vi "test add event.vi"() -> ()   [LabVIEW 2019, in "Logger.lvclass"]
uses:
  Logger_class/Logger.lvclass
  Logger_class/EventData.ctl
  TypeDef/AlarmType.ctl
panel:
  out "Set 2":set{string}(c389)
  out "Set":set{string}(c389)
  in  "new events 2":T1[](array[typedef])=[{"obj_tag"="AI0", "event_tag"="AI0.OUT_OF_RANGE_MIN", "Description"="Уровень  масла (НС очистки и охлаждения). Вне диапазона (низкий уровень)", "ALARM TYPE"=enum."Alarm", "Value DBL"=-0.000720119846917187, "Value INT"=1, "Value STR"="Alarm", "Time Stamp"=timestamp(3831935304.696055 s since 1904-01-01)}, {"obj_tag"="AI1", "event_tag"="AI1.OUT_OF_RANGE_MIN", "Description"="Уровень масла (НС подачи масла). Вне диапазона (низкий уровень)", "ALARM TYPE"=enum."Alarm", "Value DBL"=-0.0006009105573664057, "Value INT"=1, "Value STR"="Alarm", "Time Stamp"=timestamp(3831935304.696158 s since 1904-01-01)}, {"obj_tag"="AI2", "event_tag"="AI2.OUT_OF_RANGE_MIN", "Description"="Температура масла (НС очистки и охлаждения). Вне диапазона (низкий уровень)", "ALARM TYPE"=enum."Alarm", "Value DBL"=-0.00046664569044360226, "Value INT"=1, "Value STR"="Alarm", "Time Stamp"=timestamp(3831935304.696252 s since 1904-01-01)}, {"obj_tag"="AI3", "event_tag"="AI3.OUT_OF_RANGE_MIN", "Description"="Температура масла (НС подачи масла). Вне диапазона (низкий уровень)", "ALARM TYPE"=enum."Alarm", "Value DBL"=-0.0006016054301681914, "Value INT"=1, "Value STR"="Alarm", "Time Stamp"=timestamp(3831935304.696363 s since 1904-01-01)}, {"obj_tag"="AI4", "event_tag"="AI4.OUT_OF_RANGE_MIN", "Description"="Обратная связь от клапана регулировки низкого давления . Вне диапазона (низкий уровень)", "ALARM TYPE"=enum."Alarm", "Value DBL"=-0.00044842458141900095, "Value INT"=1, "Value STR"="Alarm", "Time Stamp"=timestamp(3831935304.696455 s since 1904-01-01)}, {"obj_tag"="AI5", "event_tag"="AI5.OUT_OF_RANGE_MIN", "Description"="Давление после насоса ВД. Вне диапазона (низкий уровень)", "ALARM TYPE"=enum."Alarm", "Value DBL"=-0.0004746753317086808, "Value INT"=1, "Value STR"="Alarm", "Time Stamp"=timestamp(3831935304.696545 s since 1904-01-01)}, {"obj_tag"="AI6", "event_tag"="AI6.OUT_OF_RANGE_MIN", "Description"="Давление в образце. Вне диапазона (низкий уровень)", "ALARM TYPE"=enum."Alarm", "Value DBL"=-0.0004625536617219757, "Value INT"=1, "Value STR"="Alarm", "Time Stamp"=timestamp(3831935304.696636 s since 1904-01-01)}, {"obj_tag"="AI7", "event_tag"="AI7.OUT_OF_RANGE_MIN", "Description"="Давление в камере. Вне диапазона (низкий уровень)", "ALARM TYPE"=enum."Alarm", "Value DBL"=-0.0004948266429604644, "Value INT"=1, "Value STR"="Alarm", "Time Stamp"=timestamp(3831935304.696729 s since 1904-01-01)}, {"obj_tag"="AI8", "event_tag"="AI8.OUT_OF_RANGE_MIN", "Description"="Давление  в  линии подачи воздуха в  БПВ. Вне диапазона (низкий уровень)", "ALARM TYPE"=enum."Alarm", "Value DBL"=-0.0005392985022747455, "Value INT"=1, "Value STR"="Alarm", "Time Stamp"=timestamp(3831935304.696866 s since 1904-01-01)}, {"obj_tag"="AI9", "event_tag"="AI9.OUT_OF_RANGE_MIN", "Description"="Давление  в  линии подачи воздуха после БПВ. Вне диапазона (низкий уровень)", "ALARM TYPE"=enum."Alarm", "Value DBL"=-0.00044981432702257226, "Value INT"=1, "Value STR"="Alarm", "Time Stamp"=timestamp(3831935304.69696 s since 1904-01-01)}, {"obj_tag"="DI0", "event_tag"="DI0.DI", "Description"="Автомат QF1", "ALARM TYPE"=enum."Normal", "Value DBL"=1.0, "Value INT"=1, "Value STR"="True", "Time Stamp"=timestamp(3831935304.697038 s since 1904-01-01)}, {"obj_tag"="DI1", "event_tag"="DI1.DI", "Description"="Автомат QF2", "ALARM TYPE"=enum."Normal", "Value DBL"=1.0, "Value INT"=1, "Value STR"="True", "Time Stamp"=timestamp(3831935304.697049 s since 1904-01-01)}, {"obj_tag"="DI2", "event_tag"="DI2.DI", "Description"="Автомат QF3", "ALARM TYPE"=enum."Normal", "Value DBL"=1.0, "Value INT"=1, "Value STR"="True", "Time Stamp"=timestamp(3831935304.697056 s since 1904-01-01)}, {"obj_tag"="DI3", "event_tag"="DI3.DI", "Description"="Автомат QF4", "ALARM TYPE"=enum."Normal", "Value DBL"=1.0, "Value INT"=1, "Value STR"="True", "Time Stamp"=timestamp(3831935304.697061 s since 1904-01-01)}, {"obj_tag"="DI4", "event_tag"="DI4.DI", "Description"="Автомат QF5", "ALARM TYPE"=enum."Normal", "Value DBL"=1.0, "Value INT"=1, "Value STR"="True", "Time Stamp"=timestamp(3831935304.697067 s since 1904-01-01)}, {"obj_tag"="DI5", "event_tag"="DI5.DI", "Description"="Автомат QF6", "ALARM TYPE"=enum."Normal", "Value DBL"=1.0, "Value INT"=1, "Value STR"="True", "Time Stamp"=timestamp(3831935304.697073 s since 1904-01-01)}, {"obj_tag"="DI6", "event_tag"="DI6.DI", "Description"="Автомат QF7", "ALARM TYPE"=enum."Normal", "Value DBL"=1.0, "Value INT"=1, "Value STR"="True", "Time Stamp"=timestamp(3831935304.697079 s since 1904-01-01)}, {"obj_tag"="DI7", "event_tag"="DI7.DI", "Description"="Автомат QF8", "ALARM TYPE"=enum."Normal", "Value DBL"=1.0, "Value INT"=1, "Value STR"="True", "Time Stamp"=timestamp(3831935304.697137 s since 1904-01-01)}, {"obj_tag"="DI8", "event_tag"="DI8.DI", "Description"="Автомат QF9", "ALARM TYPE"=enum."Normal", "Value DBL"=1.0, "Value INT"=1, "Value STR"="True", "Time Stamp"=timestamp(3831935304.697145 s since 1904-01-01)}, {"obj_tag"="DI10", "event_tag"="DI10.DI", "Description"="Состояние БП [G1]", "ALARM TYPE"=enum."Normal", "Value DBL"=1.0, "Value INT"=1, "Value STR"="True", "Time Stamp"=timestamp(3831935304.697152 s since 1904-01-01)}, {"obj_tag"="DI11", "event_tag"="DI11.DI", "Description"="Состояние БП [G2]", "ALARM TYPE"=enum."Normal", "Value DBL"=1.0, "Value INT"=1, "Value STR"="True", "Time Stamp"=timestamp(3831935304.697158 s since 1904-01-01)}, {"obj_tag"="DI15", "event_tag"="DI15.DI", "Description"="Кнопка аварийной остановки [SB4]", "ALARM TYPE"=enum."Normal", "Value DBL"=1.0, "Value INT"=1, "Value STR"="True", "Time Stamp"=timestamp(3831935304.697164 s since 1904-01-01)}, {"obj_tag"="STAND", "event_tag"="DO5", "Description"="Клапан KP6 Y29.1 33.7", "ALARM TYPE"=enum."Normal", "Value DBL"=1.0, "Value INT"=1, "Value STR"="True", "Time Stamp"=timestamp(3831935304.697175 s since 1904-01-01)}, {"obj_tag"="STAND", "event_tag"="DO6", "Description"="Клапан KP7 Y29.2 33.8 ", "ALARM TYPE"=enum."Normal", "Value DBL"=1.0, "Value INT"=1, "Value STR"="True", "Time Stamp"=timestamp(3831935304.697185 s since 1904-01-01)}, {"obj_tag"="STAND", "event_tag"="DO7", "Description"="Клапан KP8 Y29.3 33.9 ", "ALARM TYPE"=enum."Normal", "Value DBL"=1.0, "Value INT"=1, "Value STR"="True", "Time Stamp"=timestamp(3831935304.697191 s since 1904-01-01)}, {"obj_tag"="STAND", "event_tag"="DO8", "Description"="Клапан KP9 Y29.4  33.12 ", "ALARM TYPE"=enum."Normal", "Value DBL"=1.0, "Value INT"=1, "Value STR"="True", "Time Stamp"=timestamp(3831935304.697197 s since 1904-01-01)}, {"obj_tag"="STAND", "event_tag"="DO9", "Description"="Клапан KP10 Y29.5 33.1 ", "ALARM TYPE"=enum."Normal", "Value DBL"=1.0, "Value INT"=1, "Value STR"="True", "Time Stamp"=timestamp(3831935304.697212 s since 1904-01-01)}, {"obj_tag"="STAND", "event_tag"="DO10", "Description"="Клапан KP11 Y29.6 33.2 ", "ALARM TYPE"=enum."Normal", "Value DBL"=1.0, "Value INT"=1, "Value STR"="True", "Time Stamp"=timestamp(3831935304.697243 s since 1904-01-01)}, {"obj_tag"="STAND", "event_tag"="DO11", "Description"="Клапан KP12 Y29.7  33.13 ", "ALARM TYPE"=enum."Normal", "Value DBL"=1.0, "Value INT"=1, "Value STR"="True", "Time Stamp"=timestamp(3831935304.697255 s since 1904-01-01)}, {"obj_tag"="STAND", "event_tag"="DO12", "Description"="Клапан KP13 Y29.8  33.11 ", "ALARM TYPE"=enum."Normal", "Value DBL"=1.0, "Value INT"=1, "Value STR"="True", "Time Stamp"=timestamp(3831935304.697262 s since 1904-01-01)}, {"obj_tag"="STAND", "event_tag"="DO13", "Description"="Клапан KP14 Y29.9 33.10 ", "ALARM TYPE"=enum."Normal", "Value DBL"=1.0, "Value INT"=1, "Value STR"="True", "Time Stamp"=timestamp(3831935304.697268 s since 1904-01-01)}, {"obj_tag"="STAND", "event_tag"="DO14", "Description"="Клапан KP15 Y29.10  33.6 ", "ALARM TYPE"=enum."Normal", "Value DBL"=1.0, "Value INT"=1, "Value STR"="True", "Time Stamp"=timestamp(3831935304.697274 s since 1904-01-01)}, {"obj_tag"="STAND", "event_tag"="DO15", "Description"="Клапан KP16 Y29.11  33.5 ", "ALARM TYPE"=enum."Normal", "Value DBL"=1.0, "Value INT"=1, "Value STR"="True", "Time Stamp"=timestamp(3831935304.697279 s since 1904-01-01)}, {"obj_tag"="STAND", "event_tag"="DO16", "Description"="Клапан KP17 Y29.12  33.4 ", "ALARM TYPE"=enum."Normal", "Value DBL"=1.0, "Value INT"=1, "Value STR"="True", "Time Stamp"=timestamp(3831935304.697374 s since 1904-01-01)}, {"obj_tag"="STAND", "event_tag"="DO17", "Description"="Клапан KP18 Y29.13 33.3 ", "ALARM TYPE"=enum."Normal", "Value DBL"=1.0, "Value INT"=1, "Value STR"="True", "Time Stamp"=timestamp(3831935304.697383 s since 1904-01-01)}, {"obj_tag"="STAND", "event_tag"="DO19", "Description"="Драйверы KP20", "ALARM TYPE"=enum."Normal", "Value DBL"=1.0, "Value INT"=1, "Value STR"="True", "Time Stamp"=timestamp(3831935304.69739 s since 1904-01-01)}, {"obj_tag"="STAND", "event_tag"="DO24", "Description"="Сигнал остановки шагового драйвера 1", "ALARM TYPE"=enum."Normal", "Value DBL"=1.0, "Value INT"=1, "Value STR"="True", "Time Stamp"=timestamp(3831935304.697397 s since 1904-01-01)}, {"obj_tag"="STAND", "event_tag"="DO25", "Description"="Сигнал остановки шагового драйвера 2", "ALARM TYPE"=enum."Normal", "Value DBL"=1.0, "Value INT"=1, "Value STR"="True", "Time Stamp"=timestamp(3831935304.697403 s since 1904-01-01)}, {"obj_tag"="NV1", "event_tag"="NV1.OL", "Description"="Игольчатый клапан плавного спуска (образец). Состояние разомкнутой нагрузки", "ALARM TYPE"=enum."Normal", "Value DBL"=0.0, "Value INT"=0, "Value STR"="Normal", "Time Stamp"=timestamp(3831935304.707156 s since 1904-01-01)}, {"obj_tag"="NV1", "event_tag"="NV1.TF", "Description"="Игольчатый клапан плавного спуска (образец). Предупреждения о перегреве и отключения при перегреве", "ALARM TYPE"=enum."Normal", "Value DBL"=0.0, "Value INT"=0, "Value STR"="Normal", "Time Stamp"=timestamp(3831935304.707491 s since 1904-01-01)}, {"obj_tag"="NV1", "event_tag"="NV1.STL", "Description"="Игольчатый клапан плавного спуска (образец). Состояние остановки двигателя", "ALARM TYPE"=enum."Normal", "Value DBL"=0.0, "Value INT"=0, "Value STR"="Normal", "Time Stamp"=timestamp(3831935304.707583 s since 1904-01-01)}, {"obj_tag"="NV1", "event_tag"="NV1.OCP", "Description"="Игольчатый клапан плавного спуска (образец). Перегрузка по току", "ALARM TYPE"=enum."Normal", "Value DBL"=0.0, "Value INT"=0, "Value STR"="Normal", "Time Stamp"=timestamp(3831935304.707645 s since 1904-01-01)}, {"obj_tag"="NV1", "event_tag"="NV1.CPUV", "Description"="Игольчатый клапан плавного спуска (образец). charge pump undervoltage", "ALARM TYPE"=enum."Normal", "Value DBL"=0.0, "Value INT"=0, "Value STR"="Normal", "Time Stamp"=timestamp(3831935304.707712 s since 1904-01-01)}, {"obj_tag"="NV1", "event_tag"="NV1.UVLO", "Description"="Игольчатый клапан плавного спуска (образец). Пониженное напряжение питания", "ALARM TYPE"=enum."Normal", "Value DBL"=0.0, "Value INT"=0, "Value STR"="Normal", "Time Stamp"=timestamp(3831935304.707769 s since 1904-01-01)}, {"obj_tag"="NV1", "event_tag"="NV1.SPI_ERROR", "Description"="Игольчатый клапан плавного спуска (образец). Ошибки протокола SPI", "ALARM TYPE"=enum."Normal", "Value DBL"=0.0, "Value INT"=0, "Value STR"="Normal", "Time Stamp"=timestamp(3831935304.707827 s since 1904-01-01)}, {"obj_tag"="NV1", "event_tag"="NV1.Fault", "Description"="Игольчатый клапан плавного спуска (образец). Общая неисправность", "ALARM TYPE"=enum."Normal", "Value DBL"=0.0, "Value INT"=0, "Value STR"="Normal", "Time Stamp"=timestamp(3831935304.707885 s since 1904-01-01)}, {"obj_tag"="NV1", "event_tag"="NV1.INIT_ERROR", "Description"="Игольчатый клапан плавного спуска (образец). Ошибка инициализации", "ALARM TYPE"=enum."Normal", "Value DBL"=0.0, "Value INT"=0, "Value STR"="Normal", "Time Stamp"=timestamp(3831935304.707946 s since 1904-01-01)}, {"obj_tag"="NV1", "event_tag"="NV1.MB_ERROR", "Description"="Игольчатый клапан плавного спуска (образец). Ошибка подключения (модбас)", "ALARM TYPE"=enum."Normal", "Value DBL"=0.0, "Value INT"=0, "Value STR"="Normal", "Time Stamp"=timestamp(3831935304.707986 s since 1904-01-01)}, {"obj_tag"="NV1", "event_tag"="NV1.ST", "Description"="Игольчатый клапан плавного спуска (образец). Состояние", "ALARM TYPE"=enum."Normal", "Value DBL"=0.0, "Value INT"=0, "Value STR"="IDLE", "Time Stamp"=timestamp(3831935304.708018 s since 1904-01-01)}, {"obj_tag"="M22", "event_tag"="M22.UNPLANNED_TURN_OFF", "Description"="Двигатель охлаждения. Выключение без команды", "ALARM TYPE"=enum."Normal", "Value DBL"=0.0, "Value INT"=0, "Value STR"="Normal", "Time Stamp"=timestamp(3831935304.70986 s since 1904-01-01)}, {"obj_tag"="M12", "event_tag"="M12.UNPLANNED_TURN_OFF", "Description"="Двигатель перекачки. Выключение без команды", "ALARM TYPE"=enum."Normal", "Value DBL"=0.0, "Value INT"=0, "Value STR"="Normal", "Time Stamp"=timestamp(3831935304.71006 s since 1904-01-01)}, {"obj_tag"="M21", "event_tag"="M21.UNPLANNED_TURN_OFF", "Description"="Двигатель подачи масла. Выключение без команды", "ALARM TYPE"=enum."Normal", "Value DBL"=0.0, "Value INT"=0, "Value STR"="Normal", "Time Stamp"=timestamp(3831935304.71022 s since 1904-01-01)}, {"obj_tag"="M22", "event_tag"="M22.AUTOMAT_ERROR", "Description"="Двигатель охлаждения. Выключен автомат", "ALARM TYPE"=enum."Normal", "Value DBL"=0.0, "Value INT"=0, "Value STR"="Normal", "Time Stamp"=timestamp(3831935304.710246 s since 1904-01-01)}, {"obj_tag"="M22", "event_tag"="M22.UNPLANNED_TURN_ON", "Description"="Двигатель охлаждения. Включение без команды", "ALARM TYPE"=enum."Normal", "Value DBL"=0.0, "Value INT"=0, "Value STR"="Normal", "Time Stamp"=timestamp(3831935304.710273 s since 1904-01-01)}, {"obj_tag"="M22", "event_tag"="M22.ON_EEROR", "Description"="Двигатель охлаждения. Ошибка включения", "ALARM TYPE"=enum."Normal", "Value DBL"=0.0, "Value INT"=0, "Value STR"="Normal", "Time Stamp"=timestamp(3831935304.710294 s since 1904-01-01)}, {"obj_tag"="M22", "event_tag"="M22.OFF_ERROR", "Description"="Двигатель охлаждения. Ошибка выключения", "ALARM TYPE"=enum."Normal", "Value DBL"=0.0, "Value INT"=0, "Value STR"="Normal", "Time Stamp"=timestamp(3831935304.710315 s since 1904-01-01)}, {"obj_tag"="M22", "event_tag"="M22.ST", "Description"="Двигатель охлаждения. Состояние", "ALARM TYPE"=enum."Normal", "Value DBL"=1.0, "Value INT"=1, "Value STR"="Off", "Time Stamp"=timestamp(3831935304.710339 s since 1904-01-01)}, {"obj_tag"="M12", "event_tag"="M12.AUTOMAT_ERROR", "Description"="Двигатель перекачки. Выключен автомат", "ALARM TYPE"=enum."Normal", "Value DBL"=0.0, "Value INT"=0, "Value STR"="Normal", "Time Stamp"=timestamp(3831935304.710367 s since 1904-01-01)}, {"obj_tag"="M12", "event_tag"="M12.UNPLANNED_TURN_ON", "Description"="Двигатель перекачки. Включение без команды", "ALARM TYPE"=enum."Normal", "Value DBL"=0.0, "Value INT"=0, "Value STR"="Normal", "Time Stamp"=timestamp(3831935304.710392 s since 1904-01-01)}, {"obj_tag"="M12", "event_tag"="M12.ON_EEROR", "Description"="Двигатель перекачки. Ошибка включения", "ALARM TYPE"=enum."Normal", "Value DBL"=0.0, "Value INT"=0, "Value STR"="Normal", "Time Stamp"=timestamp(3831935304.710413 s since 1904-01-01)}, {"obj_tag"="M12", "event_tag"="M12.OFF_ERROR", "Description"="Двигатель перекачки. Ошибка выключения", "ALARM TYPE"=enum."Normal", "Value DBL"=0.0, "Value INT"=0, "Value STR"="Normal", "Time Stamp"=timestamp(3831935304.710432 s since 1904-01-01)}, {"obj_tag"="M12", "event_tag"="M12.ST", "Description"="Двигатель перекачки. Состояние", "ALARM TYPE"=enum."Normal", "Value DBL"=1.0, "Value INT"=1, "Value STR"="Off", "Time Stamp"=timestamp(3831935304.710451 s since 1904-01-01)}, {"obj_tag"="M21", "event_tag"="M21.AUTOMAT_ERROR", "Description"="Двигатель подачи масла. Выключен автомат", "ALARM TYPE"=enum."Normal", "Value DBL"=0.0, "Value INT"=0, "Value STR"="Normal", "Time Stamp"=timestamp(3831935304.710473 s since 1904-01-01)}, {"obj_tag"="M21", "event_tag"="M21.UNPLANNED_TURN_ON", "Description"="Двигатель подачи масла. Включение без команды", "ALARM TYPE"=enum."Normal", "Value DBL"=0.0, "Value INT"=0, "Value STR"="Normal", "Time Stamp"=timestamp(3831935304.710492 s since 1904-01-01)}, {"obj_tag"="M21", "event_tag"="M21.ON_EEROR", "Description"="Двигатель подачи масла. Ошибка включения", "ALARM TYPE"=enum."Normal", "Value DBL"=0.0, "Value INT"=0, "Value STR"="Normal", "Time Stamp"=timestamp(3831935304.710516 s since 1904-01-01)}, {"obj_tag"="M21", "event_tag"="M21.OFF_ERROR", "Description"="Двигатель подачи масла. Ошибка выключения", "ALARM TYPE"=enum."Normal", "Value DBL"=0.0, "Value INT"=0, "Value STR"="Normal", "Time Stamp"=timestamp(3831935304.710727 s since 1904-01-01)}, {"obj_tag"="M21", "event_tag"="M21.ST", "Description"="Двигатель подачи масла. Состояние", "ALARM TYPE"=enum."Normal", "Value DBL"=1.0, "Value INT"=1, "Value STR"="Off", "Time Stamp"=timestamp(3831935304.71075 s since 1904-01-01)}, {"obj_tag"="VALVE_44_1", "event_tag"="VALVE_44_1.LIMITS_ERROR", "Description"="Клапан 44.1. Ошибочное состояние концевиков", "ALARM TYPE"=enum."Normal", "Value DBL"=0.0, "Value INT"=0, "Value STR"="Normal", "Time Stamp"=timestamp(3831935304.711082 s since 1904-01-01)}, {"obj_tag"="VALVE_44_1", "event_tag"="VALVE_44_1.UNPLANNED_CLOSE", "Description"="Клапан 44.1. Закрытие без команды", "ALARM TYPE"=enum."Normal", "Value DBL"=0.0, "Value INT"=0, "Value STR"="Normal", "Time Stamp"=timestamp(3831935304.711128 s since 1904-01-01)}, {"obj_tag"="VALVE_44_1", "event_tag"="VALVE_44_1.UNPLANNED_OPEN", "Description"="Клапан 44.1. Открытие без команды", "ALARM TYPE"=enum."Normal", "Value DBL"=0.0, "Value INT"=0, "Value STR"="Normal", "Time Stamp"=timestamp(3831935304.711153 s since 1904-01-01)}, {"obj_tag"="VALVE_44_1", "event_tag"="VALVE_44_1.OPEN_ERROR", "Description"="Клапан 44.1. Ошибка открытия", "ALARM TYPE"=enum."Normal", "Value DBL"=0.0, "Value INT"=0, "Value STR"="Normal", "Time Stamp"=timestamp(3831935304.71118 s since 1904-01-01)}, {"obj_tag"="VALVE_44_1", "event_tag"="VALVE_44_1.CLOSE_ERROR", "Description"="Клапан 44.1.Ошибка закрытия", "ALARM TYPE"=enum."Normal", "Value DBL"=0.0, "Value INT"=0, "Value STR"="Normal", "Time Stamp"=timestamp(3831935304.711201 s since 1904-01-01)}, {"obj_tag"="VALVE_44_1", "event_tag"="VALVE_44_1.ST", "Description"="Клапан 44.1. Состояние", "ALARM TYPE"=enum."Normal", "Value DBL"=0.0, "Value INT"=0, "Value STR"="Unknown", "Time Stamp"=timestamp(3831935304.711225 s since 1904-01-01)}, {"obj_tag"="VALVE_44_2", "event_tag"="VALVE_44_2.LIMITS_ERROR", "Description"="Клапан 44.2. Ошибочное состояние концевиков", "ALARM TYPE"=enum."Normal", "Value DBL"=0.0, "Value INT"=0, "Value STR"="Normal", "Time Stamp"=timestamp(3831935304.711441 s since 1904-01-01)}, {"obj_tag"="VALVE_44_2", "event_tag"="VALVE_44_2.UNPLANNED_CLOSE", "Description"="Клапан 44.2. Закрытие без команды", "ALARM TYPE"=enum."Normal", "Value DBL"=0.0, "Value INT"=0, "Value STR"="Normal", "Time Stamp"=timestamp(3831935304.711487 s since 1904-01-01)}, {"obj_tag"="VALVE_44_2", "event_tag"="VALVE_44_2.UNPLANNED_OPEN", "Description"="Клапан 44.2. Открытие без команды", "ALARM TYPE"=enum."Normal", "Value DBL"=0.0, "Value INT"=0, "Value STR"="Normal", "Time Stamp"=timestamp(3831935304.711512 s since 1904-01-01)}, {"obj_tag"="VALVE_44_2", "event_tag"="VALVE_44_2.OPEN_ERROR", "Description"="Клапан 44.2. Ошибка открытия", "ALARM TYPE"=enum."Normal", "Value DBL"=0.0, "Value INT"=0, "Value STR"="Normal", "Time Stamp"=timestamp(3831935304.711537 s since 1904-01-01)}, {"obj_tag"="VALVE_44_2", "event_tag"="VALVE_44_2.CLOSE_ERROR", "Description"="Клапан 44.2.Ошибка закрытия", "ALARM TYPE"=enum."Normal", "Value DBL"=0.0, "Value INT"=0, "Value STR"="Normal", "Time Stamp"=timestamp(3831935304.711557 s since 1904-01-01)}, {"obj_tag"="STAND", "event_tag"="ERROR_QF1", "Description"="Ошибка автомат QF1", "ALARM TYPE"=enum."Normal", "Value DBL"=0.0, "Value INT"=0, "Value STR"="Normal", "Time Stamp"=timestamp(3831935304.711661 s since 1904-01-01)}, {"obj_tag"="STAND", "event_tag"="ERROR_QF2", "Description"="Ошибка автомат QF2", "ALARM TYPE"=enum."Normal", "Value DBL"=0.0, "Value INT"=0, "Value STR"="Normal", "Time Stamp"=timestamp(3831935304.711695 s since 1904-01-01)}, {"obj_tag"="STAND", "event_tag"="ERROR_QF3", "Description"="Ошибка автомат QF3", "ALARM TYPE"=enum."Normal", "Value DBL"=0.0, "Value INT"=0, "Value STR"="Normal", "Time Stamp"=timestamp(3831935304.711716 s since 1904-01-01)}, {"obj_tag"="STAND", "event_tag"="ERROR_QF4", "Description"="Ошибка автомат QF4", "ALARM TYPE"=enum."Normal", "Value DBL"=0.0, "Value INT"=0, "Value STR"="Normal", "Time Stamp"=timestamp(3831935304.711732 s since 1904-01-01)}, {"obj_tag"="STAND", "event_tag"="ERROR_QF5", "Description"="Ошибка автомат QF5", "ALARM TYPE"=enum."Normal", "Value DBL"=0.0, "Value INT"=0, "Value STR"="Normal", "Time Stamp"=timestamp(3831935304.711748 s since 1904-01-01)}, {"obj_tag"="STAND", "event_tag"="ERROR_QF6", "Description"="Ошибка автомат QF6", "ALARM TYPE"=enum."Normal", "Value DBL"=0.0, "Value INT"=0, "Value STR"="Normal", "Time Stamp"=timestamp(3831935304.711763 s since 1904-01-01)}, {"obj_tag"="STAND", "event_tag"="ERROR_QF7", "Description"="Ошибка автомат QF7", "ALARM TYPE"=enum."Normal", "Value DBL"=0.0, "Value INT"=0, "Value STR"="Normal", "Time Stamp"=timestamp(3831935304.711784 s since 1904-01-01)}, {"obj_tag"="STAND", "event_tag"="ERROR_QF8", "Description"="Ошибка автомат QF8", "ALARM TYPE"=enum."Normal", "Value DBL"=0.0, "Value INT"=0, "Value STR"="Normal", "Time Stamp"=timestamp(3831935304.711801 s since 1904-01-01)}, {"obj_tag"="STAND", "event_tag"="ERROR_QF9", "Description"="Ошибка автомат QF9", "ALARM TYPE"=enum."Normal", "Value DBL"=0.0, "Value INT"=0, "Value STR"="Normal", "Time Stamp"=timestamp(3831935304.711817 s since 1904-01-01)}, {"obj_tag"="STAND", "event_tag"="ERROR_QF9_FCR", "Description"="Ошибка реле контроля фаз", "ALARM TYPE"=enum."Normal", "Value DBL"=0.0, "Value INT"=0, "Value STR"="Normal", "Time Stamp"=timestamp(3831935304.711834 s since 1904-01-01)}, {"obj_tag"="STAND", "event_tag"="ERROR_G1", "Description"="Ошибка БП G1", "ALARM TYPE"=enum."Normal", "Value DBL"=0.0, "Value INT"=0, "Value STR"="Normal", "Time Stamp"=timestamp(3831935304.711856 s since 1904-01-01)}, {"obj_tag"="STAND", "event_tag"="ERROR_G2", "Description"="Ошибка БП G2", "ALARM TYPE"=enum."Normal", "Value DBL"=0.0, "Value INT"=0, "Value STR"="Normal", "Time Stamp"=timestamp(3831935304.711872 s since 1904-01-01)}, {"obj_tag"="STAND", "event_tag"="ERROR_MOD_1_NI_9425", "Description"="ERROR_MOD_1_NI_9425", "ALARM TYPE"=enum."Normal", "Value DBL"=0.0, "Value INT"=0, "Value STR"="Normal", "Time Stamp"=timestamp(3831935304.712015 s since 1904-01-01)}, {"obj_tag"="STAND", "event_tag"="ERROR_MOD_2_NI_9477", "Description"="ERROR_MOD_2_NI_9477", "ALARM TYPE"=enum."Normal", "Value DBL"=0.0, "Value INT"=0, "Value STR"="Normal", "Time Stamp"=timestamp(3831935304.712038 s since 1904-01-01)}, {"obj_tag"="STAND", "event_tag"="ERROR_MOD_3_NI_9203", "Description"="ERROR_MOD_3_NI_9203", "ALARM TYPE"=enum."Normal", "Value DBL"=0.0, "Value INT"=0, "Value STR"="Normal", "Time Stamp"=timestamp(3831935304.712056 s since 1904-01-01)}, {"obj_tag"="STAND", "event_tag"="ERROR_MOD_4_NI_9203", "Description"="ERROR_MOD_4_NI_9203", "ALARM TYPE"=enum."Normal", "Value DBL"=0.0, "Value INT"=0, "Value STR"="Normal", "Time Stamp"=timestamp(3831935304.712072 s since 1904-01-01)}, {"obj_tag"="STAND", "event_tag"="ERROR_MOD_5_NI_9263", "Description"="ERROR_MOD_5_NI_9263", "ALARM TYPE"=enum."Normal", "Value DBL"=0.0, "Value INT"=0, "Value STR"="Normal", "Time Stamp"=timestamp(3831935304.712089 s since 1904-01-01)}, {"obj_tag"="NV2", "event_tag"="NV2.OL", "Description"="Игольчатый клапан плавного спуска (камера). Состояние разомкнутой нагрузки", "ALARM TYPE"=enum."Normal", "Value DBL"=0.0, "Value INT"=0, "Value STR"="Normal", "Time Stamp"=timestamp(3831935304.721548 s since 1904-01-01)}, {"obj_tag"="NV2", "event_tag"="NV2.STL", "Description"="Игольчатый клапан плавного спуска (камера). Состояние остановки двигателя", "ALARM TYPE"=enum."Normal", "Value DBL"=0.0, "Value INT"=0, "Value STR"="Normal", "Time Stamp"=timestamp(3831935304.72169 s since 1904-01-01)}, {"obj_tag"="NV2", "event_tag"="NV2.TF", "Description"="Игольчатый клапан плавного спуска (камера). Предупреждения о перегреве и отключения при перегреве", "ALARM TYPE"=enum."Normal", "Value DBL"=0.0, "Value INT"=0, "Value STR"="Normal", "Time Stamp"=timestamp(3831935304.72174 s since 1904-01-01)}, {"obj_tag"="NV2", "event_tag"="NV2.CPUV", "Description"="Игольчатый клапан плавного спуска (камера). charge pump undervoltage", "ALARM TYPE"=enum."Normal", "Value DBL"=0.0, "Value INT"=0, "Value STR"="Normal", "Time Stamp"=timestamp(3831935304.721766 s since 1904-01-01)}, {"obj_tag"="NV2", "event_tag"="NV2.OCP", "Description"="Игольчатый клапан плавного спуска (камера). Перегрузка по току", "ALARM TYPE"=enum."Normal", "Value DBL"=0.0, "Value INT"=0, "Value STR"="Normal", "Time Stamp"=timestamp(3831935304.721877 s since 1904-01-01)}, {"obj_tag"="NV2", "event_tag"="NV2.SPI_ERROR", "Description"="Игольчатый клапан плавного спуска (камера). Ошибки протокола SPI", "ALARM TYPE"=enum."Normal", "Value DBL"=0.0, "Value INT"=0, "Value STR"="Normal", "Time Stamp"=timestamp(3831935304.721945 s since 1904-01-01)}, {"obj_tag"="NV2", "event_tag"="NV2.Fault", "Description"="Игольчатый клапан плавного спуска (камера). Общая неисправность", "ALARM TYPE"=enum."Normal", "Value DBL"=0.0, "Value INT"=0, "Value STR"="Normal", "Time Stamp"=timestamp(3831935304.721971 s since 1904-01-01)}, {"obj_tag"="NV2", "event_tag"="NV2.INIT_ERROR", "Description"="Игольчатый клапан плавного спуска (камера). Ошибка инициализации", "ALARM TYPE"=enum."Normal", "Value DBL"=0.0, "Value INT"=0, "Value STR"="Normal", "Time Stamp"=timestamp(3831935304.721998 s since 1904-01-01)}, {"obj_tag"="NV2", "event_tag"="NV2.UVLO", "Description"="Игольчатый клапан плавного спуска (камера). Пониженное напряжение питания", "ALARM TYPE"=enum."Normal", "Value DBL"=0.0, "Value INT"=0, "Value STR"="Normal", "Time Stamp"=timestamp(3831935304.722071 s since 1904-01-01)}, {"obj_tag"="NV2", "event_tag"="NV2.MB_ERROR", "Description"="Игольчатый клапан плавного спуска (камера). Ошибка подключения (модбас)", "ALARM TYPE"=enum."Normal", "Value DBL"=0.0, "Value INT"=0, "Value STR"="Normal", "Time Stamp"=timestamp(3831935304.722068 s since 1904-01-01)}, {"obj_tag"="NV2", "event_tag"="NV2.ST", "Description"="Игольчатый клапан плавного спуска (камера). Состояние", "ALARM TYPE"=enum."Normal", "Value DBL"=0.0, "Value INT"=0, "Value STR"="IDLE", "Time Stamp"=timestamp(3831935304.722119 s since 1904-01-01)}, {"obj_tag"="NV1", "event_tag"="NV1.SPI_ERROR", "Description"="Игольчатый клапан плавного спуска (образец). Ошибки протокола SPI", "ALARM TYPE"=enum."Alarm", "Value DBL"=1.0, "Value INT"=1, "Value STR"="Alarm", "Time Stamp"=timestamp(3831935305.242543 s since 1904-01-01)}, {"obj_tag"="NV1", "event_tag"="NV1.Fault", "Description"="Игольчатый клапан плавного спуска (образец). Общая неисправность", "ALARM TYPE"=enum."Alarm", "Value DBL"=1.0, "Value INT"=1, "Value STR"="Alarm", "Time Stamp"=timestamp(3831935305.242568 s since 1904-01-01)}, {"obj_tag"="NV1", "event_tag"="NV1.UVLO", "Description"="Игольчатый клапан плавного спуска (образец). Пониженное напряжение питания", "ALARM TYPE"=enum."Alarm", "Value DBL"=1.0, "Value INT"=1, "Value STR"="Alarm", "Time Stamp"=timestamp(3831935305.242488 s since 1904-01-01)}, {"obj_tag"="NV2", "event_tag"="NV2.SPI_ERROR", "Description"="Игольчатый клапан плавного спуска (камера). Ошибки протокола SPI", "ALARM TYPE"=enum."Alarm", "Value DBL"=1.0, "Value INT"=1, "Value STR"="Alarm", "Time Stamp"=timestamp(3831935305.248024 s since 1904-01-01)}, {"obj_tag"="NV2", "event_tag"="NV2.Fault", "Description"="Игольчатый клапан плавного спуска (камера). Общая неисправность", "ALARM TYPE"=enum."Alarm", "Value DBL"=1.0, "Value INT"=1, "Value STR"="Alarm", "Time Stamp"=timestamp(3831935305.248053 s since 1904-01-01)}, {"obj_tag"="NV2", "event_tag"="NV2.UVLO", "Description"="Игольчатый клапан плавного спуска (камера). Пониженное напряжение питания", "ALARM TYPE"=enum."Alarm", "Value DBL"=1.0, "Value INT"=1, "Value STR"="Alarm", "Time Stamp"=timestamp(3831935305.247993 s since 1904-01-01)}, {"obj_tag"="M22", "event_tag"="M22.AUTOMAT_ERROR", "Description"="Двигатель охлаждения. Выключен автомат", "ALARM TYPE"=enum."Alarm", "Value DBL"=1.0, "Value INT"=1, "Value STR"="Alarm", "Time Stamp"=timestamp(3831935305.303906 s since 1904-01-01)}, {"obj_tag"="M12", "event_tag"="M12.AUTOMAT_ERROR", "Description"="Двигатель перекачки. Выключен автомат", "ALARM TYPE"=enum."Alarm", "Value DBL"=1.0, "Value INT"=1, "Value STR"="Alarm", "Time Stamp"=timestamp(3831935305.303964 s since 1904-01-01)}, {"obj_tag"="M21", "event_tag"="M21.AUTOMAT_ERROR", "Description"="Двигатель подачи масла. Выключен автомат", "ALARM TYPE"=enum."Alarm", "Value DBL"=1.0, "Value INT"=1, "Value STR"="Alarm", "Time Stamp"=timestamp(3831935305.303993 s since 1904-01-01)}, {"obj_tag"="STAND", "event_tag"="ERROR_QF9_FCR", "Description"="Ошибка реле контроля фаз", "ALARM TYPE"=enum."Alarm", "Value DBL"=1.0, "Value INT"=1, "Value STR"="Alarm", "Time Stamp"=timestamp(3831935305.30444 s since 1904-01-01)}, {"obj_tag"="STAND", "event_tag"="DO24", "Description"="Сигнал остановки шагового драйвера 1", "ALARM TYPE"=enum."Normal", "Value DBL"=0.0, "Value INT"=0, "Value STR"="False", "Time Stamp"=timestamp(3831935305.49651 s since 1904-01-01)}, {"obj_tag"="STAND", "event_tag"="DO25", "Description"="Сигнал остановки шагового драйвера 2", "ALARM TYPE"=enum."Normal", "Value DBL"=0.0, "Value INT"=0, "Value STR"="False", "Time Stamp"=timestamp(3831935305.496523 s since 1904-01-01)}]
  out "CurrentEvents 2":T1[](array[typedef])
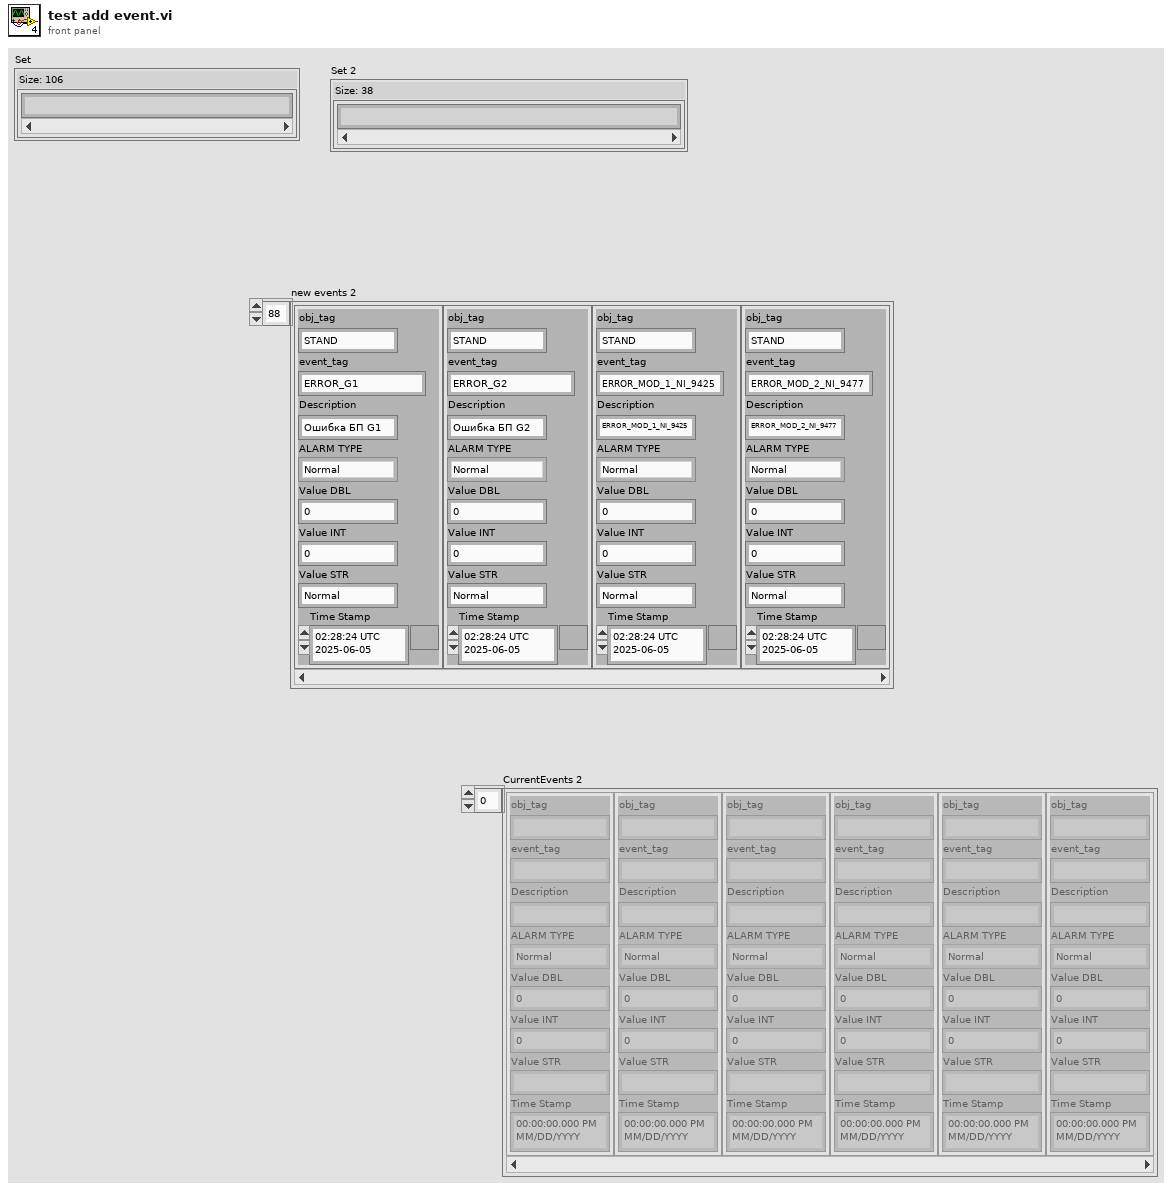
[diagram p1: front panel]
types:
  T1 = typedef "EventData.ctl" = cluster{"obj_tag":string, "event_tag":string, "Description":string, "ALARM TYPE":T2, "Value DBL":dbl, "Value INT":i32, "Value STR":string, "Time Stamp":timestamp}
  T2 = typedef "AlarmType.ctl" = enum16{"Normal", "Warning", "Alarm"}
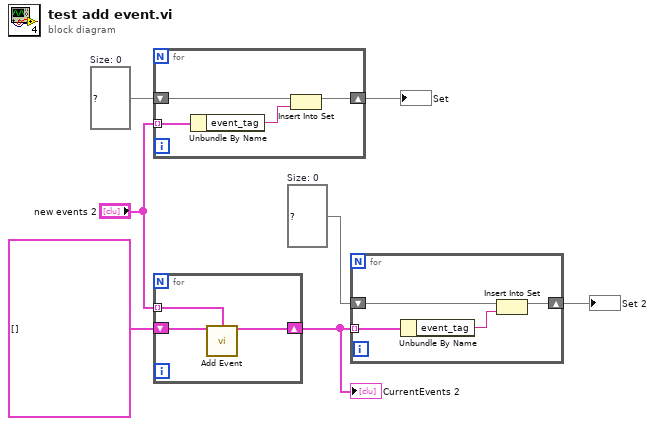
[diagram p0: block diagram]
diagram:
  w3 = set{string} {}  # Size: 0
  w6 = set{string} {}  # Size: 0
  n1 = for {
    tunnel: "new events 2" -> [w11] mode=indexing
    shift-right: [w9] -> w5
    shift-left: w6 -> [w8]
    n2 = Unbundle By Name(w11) -> ("event_tag"=w10:string)
    n3 = Insert Into Set(10:w10, 11:w8) -> (3:w9:set{string})  [unwired: 1 out]
  }
  "Set" <- w5
  n4 = for {
    tunnel: "new events 2" -> [w12] mode=indexing
    shift-right: [w14] -> w2
    shift-left: T1[] [] ("CurrentEvents out") -> [w13]
    n5 = call "Add Event.vi"("CurrentEvents In"=w13, "Event"=w12) -> ("CurrentEvents out"=w14:T1[])  [unwired: 13 in]
  }
  "CurrentEvents 2" <- w2
  n6 = for {
    tunnel: w2 -> [w18] mode=indexing
    shift-right: [w16] -> w4
    shift-left: w3 -> [w15]
    n7 = Unbundle By Name(w18) -> ("event_tag"=w17:string)
    n8 = Insert Into Set(10:w17, 11:w15) -> (3:w16:set{string})  [unwired: 1 out]
  }
  "Set 2" <- w4
